vi "Delete TreeNodeArray DVR.vi"(8 "error in (no error)":errorcluster, 11 "TreeNodeArray DVR in":refnum<data-value>) -> (0 "error out":errorcluster, 3 "TreeNodeArray out":refnum<class "TreeNodeArray.lvclass">)   [LabVIEW 2012, in "MDSplus.lvlib" / "TreeNodeArray.lvclass"]
uses:
  <vilib>/MDSplus/Classes/TreeNodeArray_Class/TreeNodeArray.lvclass
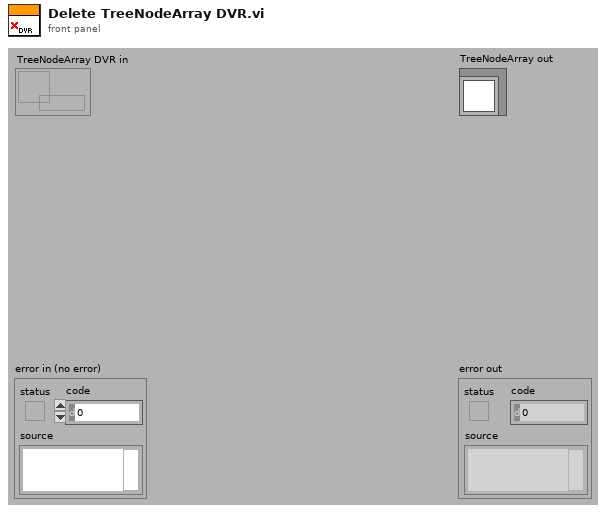
[diagram p1: front panel]
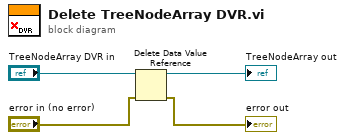
[diagram p0: block diagram]
diagram:
  n1 = Delete Data Value Reference(data value reference="TreeNodeArray DVR in", error in="error in (no error)") -> (data value=→"TreeNodeArray out":refnum<class "TreeNodeArray.lvclass">, error out=→"error out":errorcluster)
